vi "open file.vi"(8 "error in (no error)":errorcluster caption="에러 입력(에러 없음)", 10 "file path":path, 11 "Waveform File 입력":refnum<class "Waveform File.lvclass">) -> (0 "error out":errorcluster caption="에러 출력", 3 "Waveform File 출력":refnum<class "Waveform File.lvclass">)   [LabVIEW 2020, in "Waveform File.lvclass"]
uses:
  Waveform File.lvclass
  Waveform File.lvclass/Waveform File.ctl
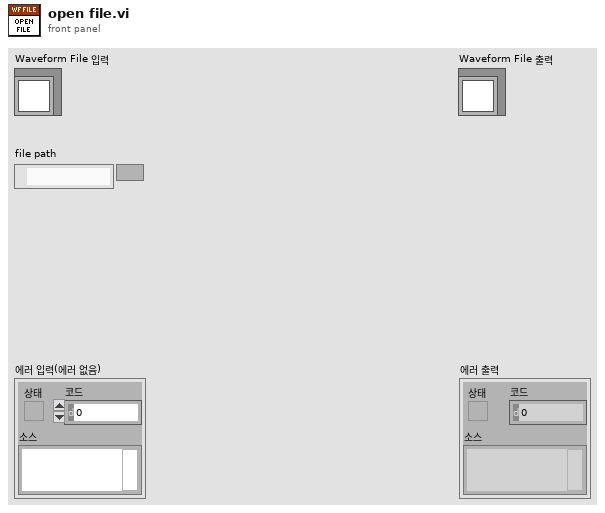
[diagram p1: front panel]
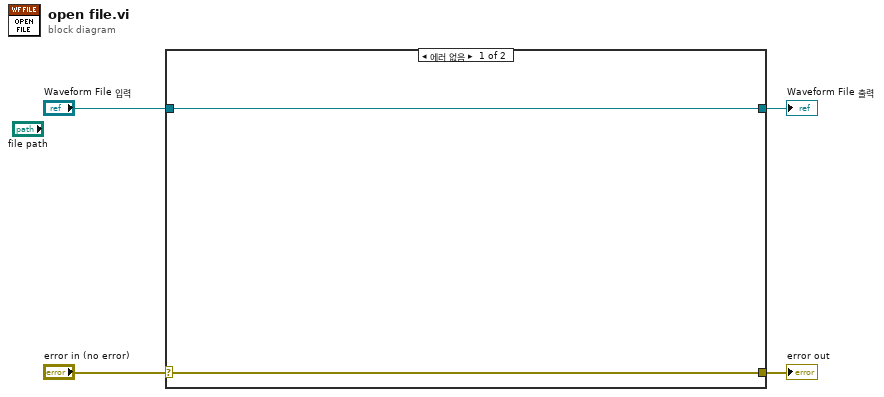
[diagram p0: block diagram]
diagram:
  n1 = case shown="에러 없음" "error in (no error)" {
    selector: "error in (no error)" -> [w5 w8]
    tunnel: [w5 w8] -> w3
    tunnel: [w6 w7] -> w1
    tunnel: "Waveform File 입력" -> [w6 w7]
    frame No Error {
    }
    frame Error {
    }
  }
  "error out" <- w3
  "Waveform File 출력" <- w1
